vi "Server Listener Stopped.vi"(8 "error in (no error)":errorcluster, 11 "Server Controller in":refnum<class "Server Controller.lvclass">) -> (0 "error out":errorcluster, 3 "Server Controller out":refnum<class "Server Controller.lvclass">)   [LabVIEW 2016, in "Server Controller.lvlib" / "Server Controller.lvclass"]
uses:
  Server Controller.lvclass
  \\Mac\Home/Documents/MAL-Framework/user.lib/Common Components/Controller/Controller.lvclass
  <vilib>/ActorFramework/Message Enqueuer/Message Enqueuer.lvclass/Message Enqueuer.ctl
  <vilib>/ActorFramework/Message Enqueuer/Enqueue.vi
  MAL-Framework/user.lib/Common Components/User Interface/Messages/Enable UI Msg/Enable UI Msg.lvclass
  C:/Program Files (x86)/National Instruments/LabVIEW 2016/vi.lib/ActorFramework/Message/Message.lvclass
  <vilib>/ActorFramework/Message Priority Queue/Priority Enqueue.vi
  MAL-Framework/user.lib/Common Components/Controller/Controller.lvclass
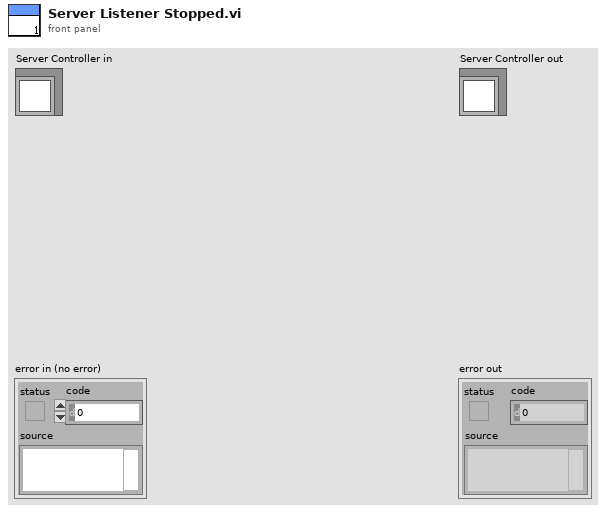
[diagram p1: front panel]
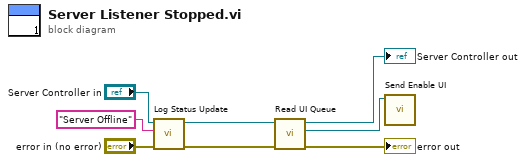
[diagram p0: block diagram]
diagram:
  n1 = call-dynamic "Log Status Update.vi"("error in (no error)"="error in (no error)", "String"="Server Offline", "Controller in"="Server Controller in") -> ("error out"=w1:errorcluster, "Controller out"=w5:refnum<class "Server Controller.lvclass">)  [unwired: 7 in]
  n2 = call "Read UI Queue.vi"("error in (no error)"=w1, "UI Controller in"=w5) -> ("error out"=→"error out":errorcluster, "UI Queue"=w7:refnum<class "Message Enqueuer.lvclass">, "UI Controller out"=→"Server Controller out":refnum<class "Server Controller.lvclass">)  [unwired: 7 in]
  n3 = call "Send Enable UI.vi"("Message Enqueuer"=w7) -> ()  [unwired: 9 in, 2 out]
